vi "Insert Table.vi"(8 "error in (no error)":errorcluster, 11 "SQLObject in":refnum<class "SQLObject.lvclass">) -> (0 "error out":errorcluster, 3 "SQLObject out":refnum<class "SQLObject.lvclass">)   [LabVIEW 2021, in "SQLObject.lvclass"]
uses:
  SQLObject.lvclass
  SQLObject.lvclass/SQLObject.ctl
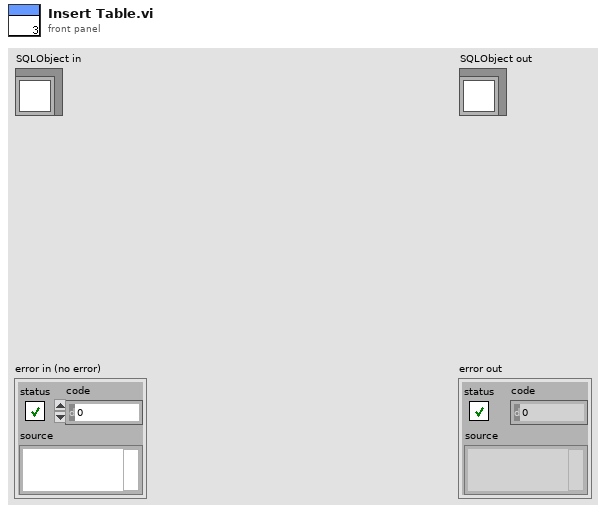
[diagram p1: front panel]
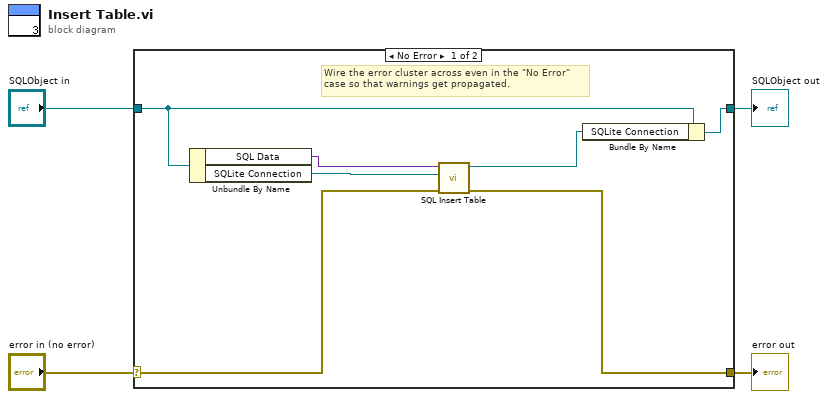
[diagram p0: block diagram]
diagram:
  n1 = case shown="No Error" "error in (no error)" {
    selector: "error in (no error)" -> [w9 w13]
    tunnel: [w8 w13] -> w3
    tunnel: [w5 w12] -> w1
    tunnel: "SQLObject in" -> [w7 w12]
    frame No Error {
      # "Wire the error cluster across even in the \"No Error\"\ncase so that warnings get propagated."
      n2 = Unbundle By Name(w7) -> ("SQL Data"=w10:variant, "SQLite Connection"=w11:refnum<class "Connection.lvclass">)
      n3 = call "SQL Insert Table.vi"("error in (no error)"=w9, "SQLite Connection in"=w11, "variant"=w10) -> ("error out"=w8:errorcluster, "SQLite Connection"=w6:refnum<class "Connection.lvclass">)  [unwired: 7 in]
      n4 = Bundle By Name(cluster=w7, "SQLite Connection"=w6) -> (w5:refnum<class "SQLObject.lvclass">)
    }
    frame Error {
    }
  }
  "error out" <- w3
  "SQLObject out" <- w1
